vi "数组索引.vi"() -> ()   [LabVIEW 2023]
doc: "本VI是为《我和LabVIEW》一书编写的示例。\n关于本书的介绍请参考网页：\nhttp://ruanqizhen.spaces.live.com/blog/cns!5852D4F797C53FB6!4310.entry"
panel:
  out "元素":string
  out "第一列":string[](array[string])
  out "第一行":string[](array[string])
  out "元素 3":string
  out "元素 2":string
  out "元素 1":string
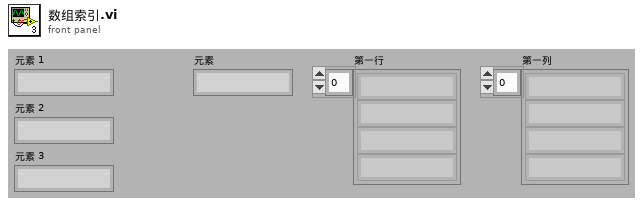
[diagram p1: front panel]
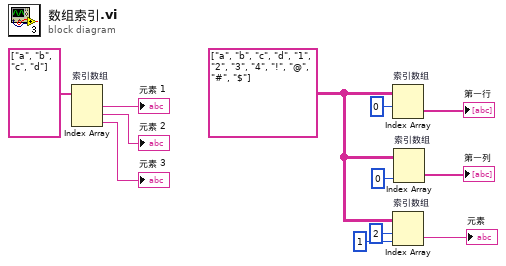
[diagram p0: block diagram]
diagram:
  w3 = string[][] [["a", "b", "c", "d"], ["1", "2", "3", "4"], ["!", "@", "#", "$"]] ("数组")
  n1 = Index Array "索引数组"(array=string[] ["a", "b", "c", "d"] ("数组")) -> (element #1=→"元素 1":string, element #2=→"元素 2":string, element #3=→"元素 3":string)  [unwired: 3 in]
  n2 = Index Array "索引数组"(array=w3, index (row)=0 ("索引 (行)")) -> (element=→"第一行":string[])  [unwired: 1 in]
  n3 = Index Array "索引数组"(array=w3, index (row)=2 ("禁用的索引 (行)"), index (col)=1 ("禁用的索引 (列)")) -> (element=→"元素":string)
  n4 = Index Array "索引数组"(array=w3, index (col)=0 ("禁用的索引 (列)")) -> (element=→"第一列":string[])  [unwired: 1 in]
